vi "Digital IOs Native.vi"() -> ()   [LabVIEW 2015]
uses:
  <vilib>/Instr/_visa.llb/VISA Configure Serial Port (Instr).vi
panel:
  out "String":string
  in  "Stop Button":bool
  in  "Baudrate":string(combo)
  out "I5":bool
  out "I4":bool
  out "I3":bool
  out "I2":bool
  out "I1":bool
  out "I0":bool
  in  "O5":bool
  in  "O4":bool
  in  "O3":bool
  in  "O2":bool
  in  "O1":bool
  in  "O0":bool
  in  "Connect":bool
  in  "VISA resource name":refnum<visa-resource-name>
  # "Digital IO LabVIEW-Proteus Simulation"
  # "Native Serial Communication"
  # "COM PORT"
  # "Outputs"
  # "Inputs"
  # "END Program"
  # "String"
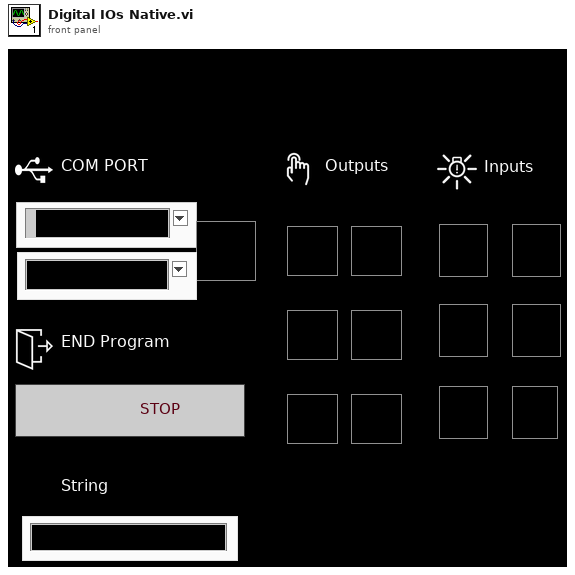
[diagram p1: front panel]
types:
  T1 = enum16{"Read Digital Values", "Write Digital Values"}
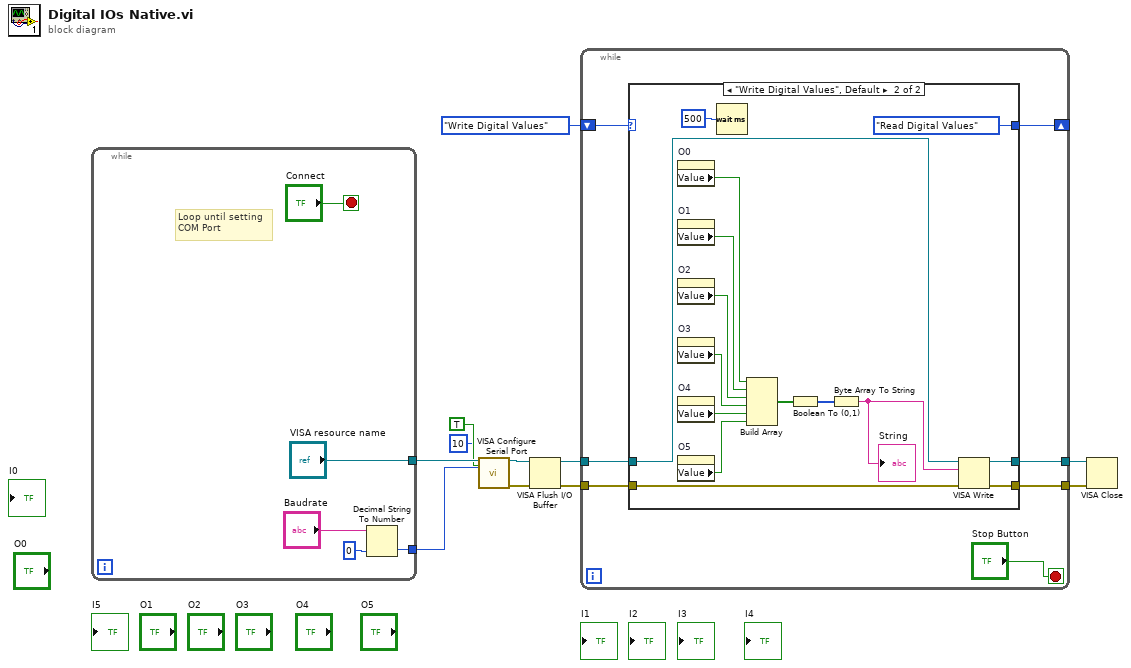
[diagram p0: block diagram]
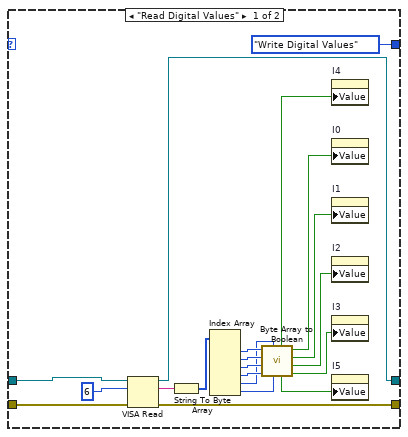
[diagram p2: hidden frame]
diagram:
  n1 = while {
    tunnel: ["VISA resource name"] -> w11
    tunnel: [w12] -> w10
    stop <- "Connect" stop-if-true
    # "Loop until setting\nCOM Port"
    n2 = Decimal String To Number(string="Baudrate", default (0L)=u32 0 ("default (0 I32)")) -> (number=w12:u32)  [unwired: 1 in, 1 out]
  }
  n3 = call-poly "VISA Configure Serial Port"("VISA resource name"=w11, "termination char\n(0xA = '\\n' = LF)"=u8 10 ("termination char\n(0xA = '\\n' = LF)"), "Enable Termination\nChar (T)"=TRUE ("Enable Termination\nChar (T)"), "baud rate (9600)"=w10) -> ("VISA resource name out"=w5:refnum<visa-resource-name>, "error out"=w4:errorcluster)  [unwired: 10 in]
  n4 = VISA Flush I/O Buffer(VISA resource name=w5, error in (no error)=w4) -> (VISA resource name out=w3:refnum<visa-resource-name>, error out=w2:errorcluster)  [unwired: 1 in]
  n5 = while {
    shift-right: [w18] -> _
    shift-left: T1."Write Digital Values" -> [w23]
    tunnel: w3 -> [w22]
    tunnel: w2 -> [w21]
    tunnel: [w20] -> w7
    tunnel: [w19] -> w6
    stop <- "Stop Button" stop-if-true
    n6 = case shown="\"Write Digital Values\", Default" w23 {
      tunnel: w22 -> [w42 w52]
      tunnel: w21 -> [w41 w51]
      tunnel: [w40 w50] -> w20
      tunnel: [w39 w49] -> w19
      tunnel: [T1."Write Digital Values" T1."Read Digital Values"] -> w18
      frame "Read Digital Values" {
        n7 = VISA Read(VISA resource name=w42, byte count=u32 6, error in (no error)=w41) -> (VISA resource name out=w40:refnum<visa-resource-name>, read buffer=w38:string, error out=w39:errorcluster)  [unwired: 1 out]
        n8 = String To Byte Array(string=w38) -> (unsigned byte array=w36:u8[])
        n9 = Index Array(array=w36) -> (element #1=w35:u8, element #2=w34:u8, element #3=w33:u8, element #4=w32:u8, element #5=w31:u8, element #6=w30:u8)  [unwired: 6 in]
        n10 = call "Byte Array to Boolean.vi"("Data 5"=w30, "Data 4"=w31, "Data 3"=w32, "Data 2"=w33, "Data 1"=w34, "Data 0"=w35) -> ("In3"=w26:bool, "In2"=w27:bool, "In1"=w28:bool, "In0"=w29:bool, "In5"=w24:bool, "In4"=w25:bool)
        n11 = property on="I4" class="Bool (strict)"("Value"=w25) -> ()  [unwired: 2 in, 2 out]
        n12 = property on="I0" class="Bool (strict)"("Value"=w29) -> ()  [unwired: 2 in, 2 out]
        n13 = property on="I1" class="Bool (strict)"("Value"=w28) -> ()  [unwired: 2 in, 2 out]
        n14 = property on="I2" class="Bool (strict)"("Value"=w27) -> ()  [unwired: 2 in, 2 out]
        n15 = property on="I3" class="Bool (strict)"("Value"=w26) -> ()  [unwired: 2 in, 2 out]
        n16 = property on="I5" class="Bool (strict)"("Value"=w24) -> ()  [unwired: 2 in, 2 out]
      }
      frame "Write Digital Values", Default {
        n17 = property on="O0" class="Bool (strict)"() -> ("Value"=w58:bool)  [unwired: 2 in, 2 out]
        n18 = property on="O1" class="Bool (strict)"() -> ("Value"=w57:bool)  [unwired: 2 in, 2 out]
        n19 = property on="O2" class="Bool (strict)"() -> ("Value"=w56:bool)  [unwired: 2 in, 2 out]
        n20 = property on="O3" class="Bool (strict)"() -> ("Value"=w55:bool)  [unwired: 2 in, 2 out]
        n21 = property on="O4" class="Bool (strict)"() -> ("Value"=w54:bool)  [unwired: 2 in, 2 out]
        n22 = property on="O5" class="Bool (strict)"() -> ("Value"=w53:bool)  [unwired: 2 in, 2 out]
        n23 = Wait (ms)(milliseconds to wait=u32 500) -> ()  [unwired: 1 out]
        n24 = Build Array(w58, w57, w56, w55, w54, w53) -> (w46:bool[])
        n25 = Boolean To (0,1)(Boolean=w46) -> (0, 1=w45:i16[])
        n26 = Byte Array To String(unsigned byte array=w45) -> (string=w44:string)
        "String" <- w44
        n27 = VISA Write(VISA resource name=w52, write buffer=w44, error in (no error)=w51) -> (VISA resource name out=w50:refnum<visa-resource-name>, error out=w49:errorcluster)  [unwired: 1 out]
      }
    }
  }
  n28 = VISA Close(VISA resource name=w7, error in (no error)=w6) -> ()  [unwired: 1 out]
